vi "NotifyIdle.vi"(8 "error in (no error)":errorcluster, 11 "BaseDriver in":refnum<class "BaseDriver.lvclass">) -> (0 "error out":errorcluster, 3 "BaseDriver out":refnum<class "BaseDriver.lvclass">)   [LabVIEW 2013, in "BaseDriver.lvclass"]
doc: "Checks if driver is Idle (nothing to send and not waiting for any response) If driver is configured for sending \"Idle\" messages, send it"
uses:
  BaseDriver.lvclass
  BaseDriver.lvclass/BaseDriver.ctl
  response.ctl
  driver_status.ctl
  Responder/BaseResponder/BaseResponder.lvclass
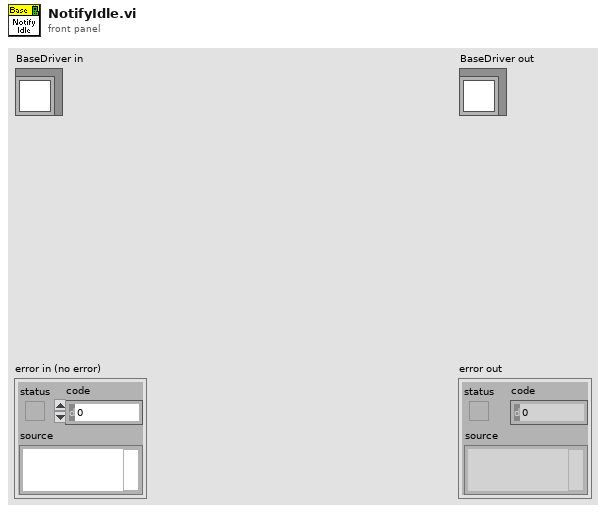
[diagram p1: front panel]
types:
  T1 = typedef "driver_status.ctl" = enum16{"Normal", "Startup", "Connection lost", "Reconnected", "Timeout", "Idle", "Busy"}
  T2 = typedef "response.ctl" = cluster{"driver status":T1, "Sender":string, "Type":i32, "Variant":variant}
  T3 = typedef "message_queue.ctl" = refnum<queue>
  T4 = typedef "driver_state.ctl" = enum16{"Idle", "Wait for ack"}
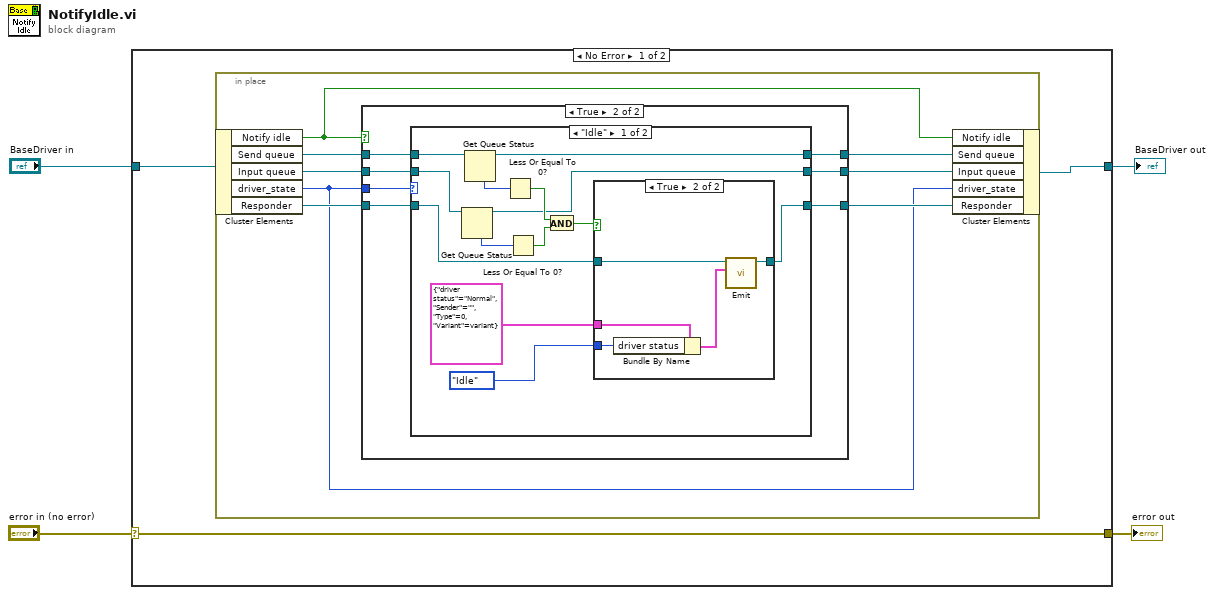
[diagram p0: block diagram]
diagram:
  n1 = case shown="No Error" "error in (no error)" {
    selector: "error in (no error)" -> [w5 w49]
    tunnel: [w5 w49] -> w3
    tunnel: [w6 w48] -> w1
    tunnel: "BaseDriver in" -> [w7 w48]
    frame No Error {
      n2 = in-place "In Place Element Structure" {
        n3 = in-place-cluster #1(w7) -> ("Notify idle"=w9:bool, "Send queue"=w15:T3, "Input queue"=w10:T3, "driver_state"=w11:T4, "Responder"=w13:refnum<class "BaseResponder.lvclass">)
        n4 = case shown="True" w9 {
          tunnel: w15 -> [w18 w25]
          tunnel: [w18 w24] -> w14
          tunnel: w11 -> [_ w23]
          tunnel: w13 -> [w17 w22]
          tunnel: [w17 w21] -> w12
          tunnel: w10 -> [w16 w20]
          tunnel: [w16 w19] -> w8
          frame False {
          }
          frame True {
            n5 = case shown="\"Idle\"" w23 {
              tunnel: w25 -> [w38 w47]
              tunnel: [w37 w47] -> w24
              tunnel: w22 -> [w35 w46]
              tunnel: [w32 w46] -> w21
              tunnel: w20 -> [w31 w45]
              tunnel: [w26 w45] -> w19
              frame "Idle" {
                n6 = Get Queue Status(queue=w31) -> (queue out=w26:T3, # elements in queue=w30:i32)  [unwired: 2 in, 6 out]
                n7 = Get Queue Status(queue=w38) -> (queue out=w37:T3, # elements in queue=w36:i32)  [unwired: 2 in, 6 out]
                n8 = Less Or Equal To 0?(x=w36) -> (x <= 0?=w29:bool)
                n9 = Less Or Equal To 0?(x=w30) -> (x <= 0?=w28:bool)
                n10 = And(x=w29, y=w28) -> (x .and. y?=w27:bool)
                n11 = case shown="True" w27 {
                  tunnel: w35 -> [w39 w44]
                  tunnel: [w39 w43] -> w32
                  tunnel: T2 {"driver status"=enum."Normal", "Sender"="", "Type"=0, "Variant"=variant} ("response") -> [_ w42]
                  tunnel: driver_status."Idle" ("driver status") -> [_ w40]
                  frame False {
                  }
                  frame True {
                    n12 = Bundle By Name(cluster=w42, "driver status"=w40) -> (w41:T2)
                    n13 = call-dynamic "Emit.vi"("response"=w41, "BaseResponder in"=w44) -> ("BaseResponder out"=w43:refnum<class "BaseResponder.lvclass">)  [unwired: 8 in, 1 out]
                  }
                }
              }
              frame "Wait for ack", Default {
              }
            }
          }
        }
        n14 = in-place-cluster #1("Notify idle"=w9, "Send queue"=w14, "Input queue"=w8, "driver_state"=w11, "Responder"=w12) -> (w6:refnum<class "BaseDriver.lvclass">)
      }
    }
    frame Error {
    }
  }
  "error out" <- w3
  "BaseDriver out" <- w1
